vi "Get Valid Routes.vi"(10 "Starting Route":T1[](array[typedef]), 11 "All Caves":T1[](array[typedef])) -> (3 "Ended Valid Routes Out":T1[][](array[typedef]))   [LabVIEW 2019, in "Day 12.lvlib"]
uses:
  Controls/Cave.ctl
  Controls/Cave Type.ctl
  Day 12.lvlib
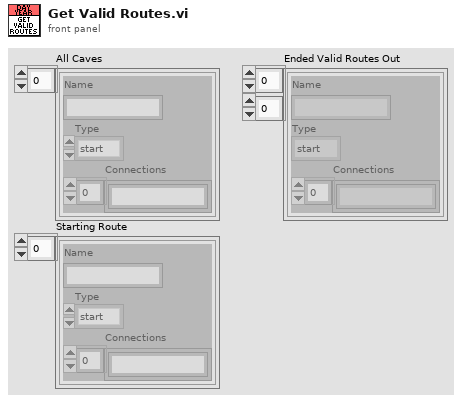
[diagram p1: front panel]
types:
  T1 = typedef "Day 12.lvlib/Cave.ctl" = cluster{"Name":string, "Type":T2, "Connections":string[]}
  T2 = typedef "Day 12.lvlib/Cave Type.ctl" = enum16{"start", "end", "small", "big"}
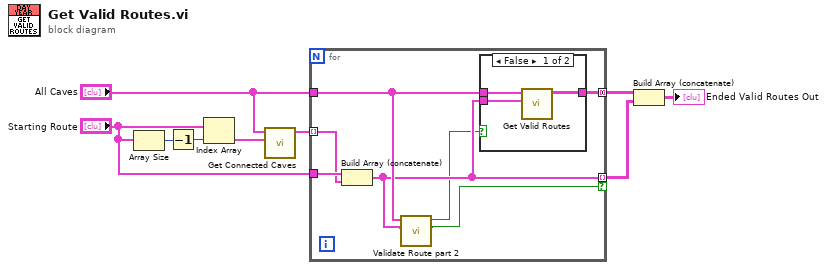
[diagram p0: block diagram]
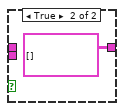
[diagram p2: hidden frame]
diagram:
  n1 = Array Size(array="Starting Route") -> (size(s)=w2:i32)
  n2 = Decrement(x=w2) -> (x-1=w1:i32)
  n3 = Index Array(array="Starting Route", index=w1) -> (element=w6:T1)
  n4 = call "Get Connected Caves.vi"("Cave"=w6, "All Caves"="All Caves") -> ("Connected Caves"=w8:T1[])  [unwired: 9 in]
  n5 = for {
    tunnel: w8 -> [w15] mode=indexing
    tunnel: "Starting Route" -> [w16]
    tunnel: "All Caves" -> [w13]
    tunnel: [w12] -> w4 mode=indexing if=w10
    tunnel: [w14] -> w5 mode=concatenating
    n6 = Build Array (concatenate)(w16, w15) -> (w12:T1[])
    n7 = call "Validate Route part 2.vi"("Path"=w12, "All Caves"=w13) -> ("End?"=w10:bool, "Invalid Path?"=w11:bool)  [unwired: 8 in]
    n8 = case shown="False" w11 {
      tunnel: w13 -> [w19 _]
      tunnel: w12 -> [w18 _]
      tunnel: [w17 T1[][] [] ("Ended Valid Routes Out")] -> w14
      frame False {
        n9 = call "Get Valid Routes.vi"("Starting Route"=w18, "All Caves"=w19) -> ("Ended Valid Routes Out"=w17:T1[][])  [unwired: 9 in]
      }
      frame True {
      }
    }
  }
  n10 = Build Array (concatenate)(w5, w4) -> (→"Ended Valid Routes Out":T1[][])
